vi "uTTA_CalReadData.vi"(7 "Control Queue":refnum<queue>, 8 "error in":errorcluster, 10 "Averaged Values":i32, 11 "Data Queue in":refnum<queue>) -> (0 "error out":errorcluster, 1 "Temp_Values":dbl[](array[numeric]), 2 "ADC_Variance":dbl[](array[numeric]), 3 "ADC_Values":dbl[](array[numeric]), 4 "Temp_Variance":dbl[](array[numeric]))   [LabVIEW 2021]
uses:
  <vilib>/Analysis/NI_AALBase.lvlib
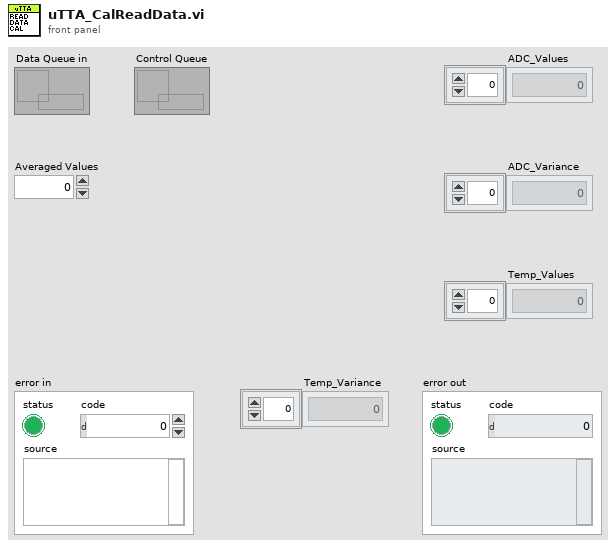
[diagram p1: front panel]
types:
  T1 = cluster{"ADC Values":i16[][], "Temperatures":dbl[][]}
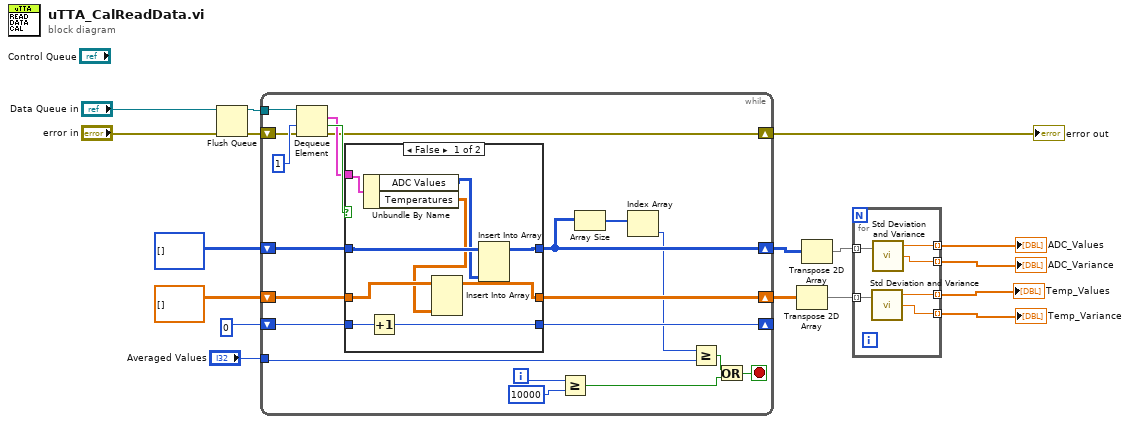
[diagram p0: block diagram]
diagram:
  n1 = Flush Queue(queue="Data Queue in", error in (no error)="error in") -> (queue out=w6:refnum<queue>, error out=w5:errorcluster)  [unwired: 1 out]
  n2 = while {
    tunnel: w6 -> [w36]
    tunnel: "Averaged Values" -> [w29]
    shift-right: [w21] -> w12
    shift-left: i32[][] [] ("ADCs") -> [w33]
    shift-right: [w31] -> w13
    shift-left: dbl[][] [] ("Temperatures") -> [w32]
    shift-right: [w19] -> _
    shift-left: 0 ("Averaged Values") -> [w30]
    shift-right: [w23] -> w1
    shift-left: w5 -> [w22]
    i -> [w25]
    stop <- w27 stop-if-true
    n3 = Dequeue Element(queue=w36, timeout in ms (-1)=1, error in (no error)=w22) -> (element=w34:T1, timed out?=w35:bool, error out=w23:errorcluster)  [unwired: 1 out]
    n4 = case shown="False" w35 {
      tunnel: w34 -> [w46 _]
      tunnel: w33 -> [w43 w49]
      tunnel: [w42 w49] -> w21
      tunnel: [w39 w48] -> w31
      tunnel: w32 -> [w40 w48]
      tunnel: w30 -> [w45 w47]
      tunnel: [w44 w47] -> w19
      frame False {
        n5 = Unbundle By Name(w46) -> ("ADC Values"=w41:i16[][], "Temperatures"=w38:dbl[][])
        n6 = Increment(x=w45) -> (x+1=w44:i32)
        n7 = Insert Into Array(array=w40, new element=w38) -> (w39:dbl[][])  [unwired: 2 in]
        n8 = Insert Into Array(array=w43, new element=w41) -> (w42:i32[][])  [unwired: 2 in]
      }
      frame True {
      }
    }
    n9 = Greater Or Equal?(x=w25, y=10000) -> (x >= y?=w26:bool)
    n10 = Array Size(array=w21) -> (size(s)=w20:i32[])
    n11 = Index Array(array=w20) -> (element=w18:i32)  [unwired: 1 in]
    n12 = Greater Or Equal?(x=w18, y=w29) -> (x >= y?=w28:bool)
    n13 = Or(x=w28, y=w26) -> (x .or. y?=w27:bool)
  }
  "error out" <- w1
  n14 = Transpose 2D Array(2D array=w13) -> (transposed array=w3:dbl[][])
  n15 = Transpose 2D Array(2D array=w12) -> (transposed array=w4:i32[][])
  n16 = for {
    tunnel: w4 -> [w55] mode=indexing
    tunnel: w3 -> [w54] mode=indexing
    tunnel: [w53] -> w16 mode=indexing
    tunnel: [w52] -> w14 mode=indexing
    tunnel: [w51] -> w15 mode=indexing
    tunnel: [w50] -> w17 mode=indexing
    n17 = call <vilib>:"Std Deviation and Variance.vi"("X"=w54) -> ("mean"=w53:dbl, "standard deviation"=w50:dbl)  [unwired: 1 in, 1 out]
    n18 = call <vilib>:"Std Deviation and Variance.vi"("X"=w55) -> ("mean"=w52:dbl, "standard deviation"=w51:dbl)  [unwired: 1 in, 1 out]
  }
  "Temp_Variance" <- w17
  "Temp_Values" <- w16
  "ADC_Variance" <- w15
  "ADC_Values" <- w14
